vi "configDotNetMember.vi"(0 "dotNetModule":refnum<k7>, 5 "Index array":i32[](array[numeric]), 7 "Parameter Value array":string[](array[string]), 11 "error in (no error)":errorcluster) -> (15 "error out":errorcluster)   [LabVIEW 2010]
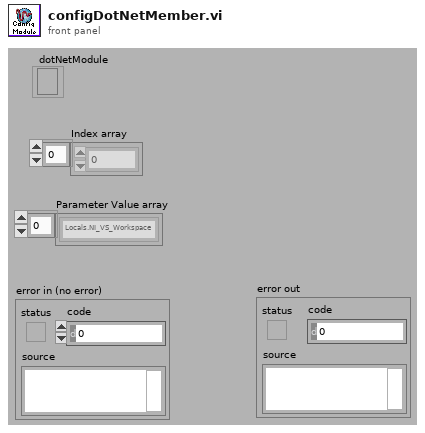
[diagram p1: front panel]
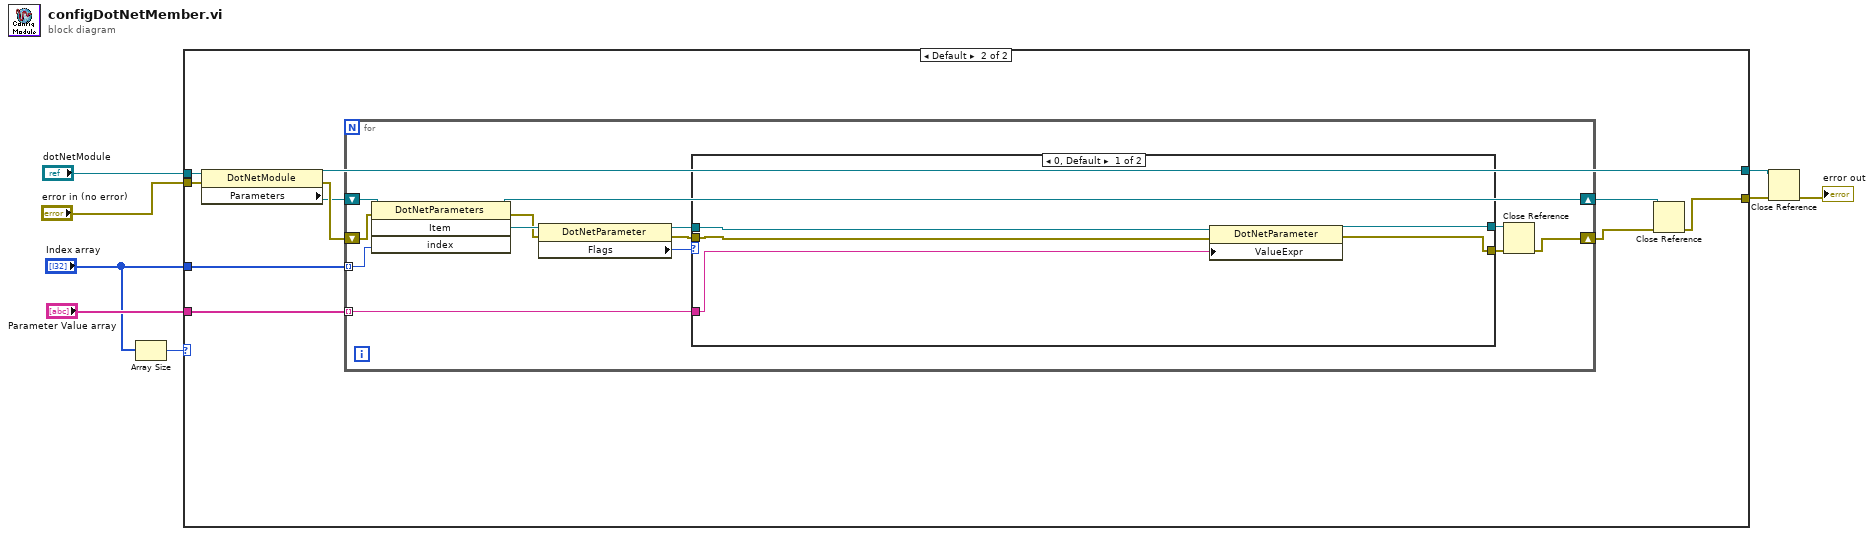
[diagram p0: block diagram]
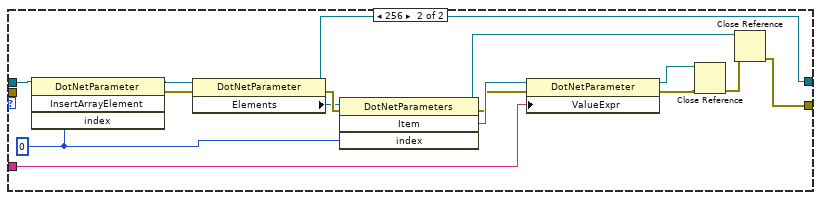
[diagram p3: hidden frame]
diagram:
  n1 = Array Size(array="Index array") -> (size(s)=w4:i32)
  n2 = case shown="Default" w4 {
    tunnel: "error in (no error)" -> [w10 w19]
    tunnel: "dotNetModule" -> [w9 w16]
    tunnel: "Parameter Value array" -> [_ w15]
    tunnel: [w10 w11] -> w3
    tunnel: "Index array" -> [_ w13]
    tunnel: [w9 w12] -> w1
    frame 0 {
    }
    frame Default {
      n3 = property class="DotNetModule"(reference=w16, error in=w19) -> (reference out=w12:refnum<k7>, error out=w20:errorcluster, "Parameters"=w17:refnum<k7>)
      n4 = for {
        tunnel: w13 -> [w31] mode=indexing
        tunnel: w15 -> [w30] mode=indexing
        shift-right: [w27] -> w14
        shift-left: w20 -> [w33]
        shift-right: [w32] -> w18
        shift-left: w17 -> [w21]
        n5 = invoke class="DotNetParameters" method="Item"(reference=w21, error in=w33, "index"=w31) -> (reference out=w32:refnum<k7>, error out=w25:errorcluster, "Item"=w26:refnum<k7>)  [unwired: 1 in, 1 out]
        n6 = property class="DotNetParameter"(reference=w26, error in=w25) -> (reference out=w23:refnum<k7>, error out=w22:errorcluster, "Flags"=w24:i32)
        n7 = case shown="0, Default" w24 {
          tunnel: w30 -> [w38 w53]
          tunnel: [w37 w44] -> w29
          tunnel: [w36 w45] -> w28
          tunnel: w23 -> [w35 w42]
          tunnel: w22 -> [w34 _]
          frame 0, Default {
            n8 = property class="DotNetParameter"(reference=w35, error in=w34, "ValueExpr"=w38) -> (reference out=w37:refnum<k7>, error out=w36:errorcluster)
          }
          frame 256 {
            w41 = 0
            n9 = invoke class="DotNetParameter" method="InsertArrayElement"(reference=w42, "index"=w41) -> (reference out=w43:refnum<k7>, error out=w40:errorcluster)  [unwired: 2 in, 2 out]
            n10 = property class="DotNetParameter"(reference=w43, error in=w40) -> (reference out=w44:refnum<k7>, error out=w50:errorcluster, "Elements"=w49:refnum<k7>)
            n11 = invoke class="DotNetParameters" method="Item"(reference=w49, error in=w50, "index"=w41) -> (reference out=w46:refnum<k7>, error out=w39:errorcluster, "Item"=w52:refnum<k7>)  [unwired: 1 in, 1 out]
            n12 = property class="DotNetParameter"(reference=w52, error in=w39, "ValueExpr"=w53) -> (reference out=w48:refnum<k7>, error out=w51:errorcluster)
            n13 = Close Reference(reference=w48, error in (no error)=w51) -> (error out=w47:errorcluster)
            n14 = Close Reference(reference=w46, error in (no error)=w47) -> (error out=w45:errorcluster)
          }
        }
        n15 = Close Reference(reference=w29, error in (no error)=w28) -> (error out=w27:errorcluster)
      }
      n16 = Close Reference(reference=w18, error in (no error)=w14) -> (error out=w11:errorcluster)
    }
  }
  n17 = Close Reference(reference=w1, error in (no error)=w3) -> (error out=→"error out":errorcluster)
